vi "K_S30_VISA F100.vi"(4 "error in":errorcluster, 6 "Index":u8=2, 7 "Address":u8=250) -> (0 "error out":errorcluster, 2 "para 0..4":u8[](array[numeric]))   [LabVIEW 2012]
panel:
  # "Function 100: Read configuration\nV1.0, b.v.\nInstead of this function you can use Function F32 if the\nTransmitter has firmware earlier 5.20-5.50."
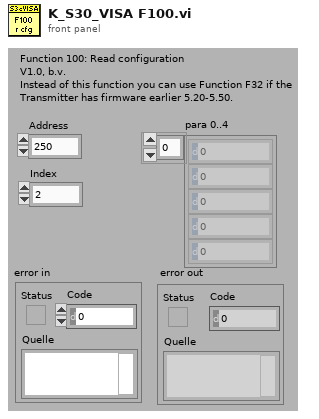
[diagram p1: front panel]
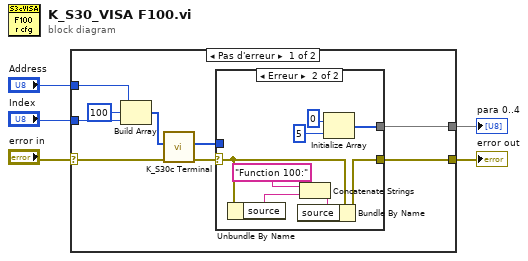
[diagram p0: block diagram]
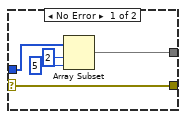
[diagram p2: hidden frame]
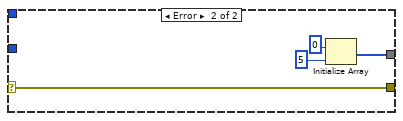
[diagram p3: hidden frame]
diagram:
  n1 = case shown="Pas d'erreur" "error in" {
    selector: "error in" -> [w11 w31]
    tunnel: "Address" -> [w14 _]
    tunnel: [w9 w31] -> w3
    tunnel: "Index" -> [w7 _]
    tunnel: [w6 w29] -> w1
    frame No Error {
      n2 = Build Array(w14, u8 100 ("Element"), w7) -> (w12:u8[])
      n3 = call "K_S30c Terminal.vi"("error in"=w11, "request"=w12) -> ("error out"=w10:errorcluster, "response"=w8:u8[])  [unwired: 4 in]
      n4 = case shown="Erreur" w10 {
        selector: w10 -> [w19 w27]
        tunnel: [w19 w25] -> w9
        tunnel: w8 -> [w18 _]
        tunnel: [w15 w20] -> w6
        frame No Error {
          n5 = Array Subset(array=w18, index=2 ("Index"), length=5 ("Länge")) -> (w15:u8[])
        }
        frame Error {
          n6 = Unbundle By Name(w27) -> ("source"=w24:string)
          n7 = Concatenate Strings("Function 100:" ("String"), w24) -> (w26:string)
          n8 = Bundle By Name(cluster=w27, "source"=w26) -> (w25:errorcluster)
          n9 = Initialize Array(u8 0, 5 ("Dimensionsgröße")) -> (w20:u8[])
        }
      }
    }
    frame Error {
      n10 = Initialize Array(u8 0, 5 ("Dimensionsgröße")) -> (w29:u8[])
    }
  }
  "error out" <- w3
  "para 0..4" <- w1
